vi "Execute.vi"(8 "error in (no error)":errorcluster, 10 "Abstract Consumer in":refnum<class "Abstract Consumer.lvclass">, 11 "Test UI Message in":refnum<class "Test UI Message.lvclass">) -> (0 "error out":errorcluster, 1 "Abstract Response out":refnum<class "Abstract Response Message.lvclass">, 2 "Abstract Consumer out":refnum<class "Abstract Consumer.lvclass">, 3 "Test UI Message out":refnum<class "Test UI Message.lvclass">, 4 "Stop?":bool)   [LabVIEW 2027, in "Test UI Message.lvclass"]
uses:
  Test UI Message.lvclass
  Consumer/Abstract Consumer/Abstract Consumer.lvclass
  Message/Abstract Response Message/Abstract Response Message.lvclass
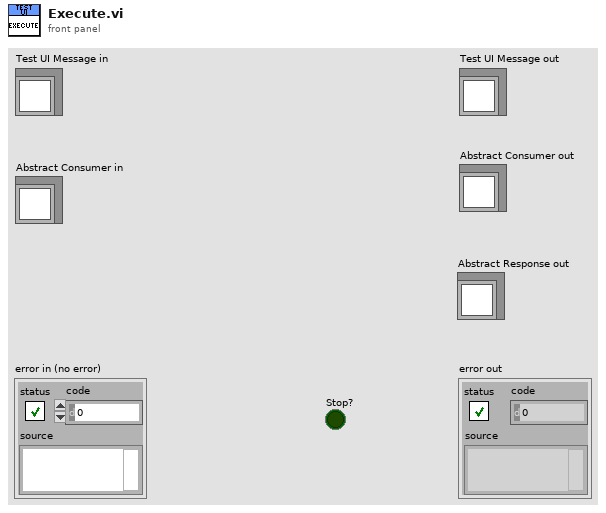
[diagram p1: front panel]
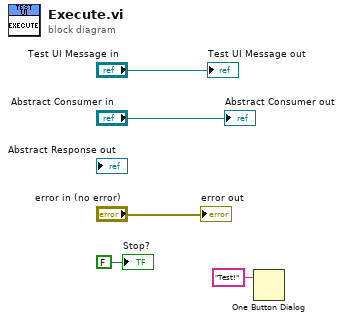
[diagram p0: block diagram]
diagram:
  n1 = One Button Dialog(message="Test!") -> ()  [unwired: 1 in, 1 out]
  "error out" <- "error in (no error)"
  "Test UI Message out" <- "Test UI Message in"
  "Abstract Consumer out" <- "Abstract Consumer in"
  "Stop?" <- FALSE ("Stop?")
